vi "Check and Generate Path to Octave Executable.vi"(8 "error in (no error)":errorcluster, 11 "octave executable file or directory with executable":path=path "C:/Octave/Octave-4.0.0/bin") -> (0 "error out":errorcluster, 3 "path to exe":path)   [LabVIEW 2020, in "GOLPI library.lvlib"]
doc: "Checks path provided by user if exists. If file, consider it as Octave executable. If directory, try to look for octave-cli.exe or octave.exe. Return path to Octave executable or generate an error."
uses:
  GOLPI library.lvlib
  Custom Error Codes Enum Type Def.vi
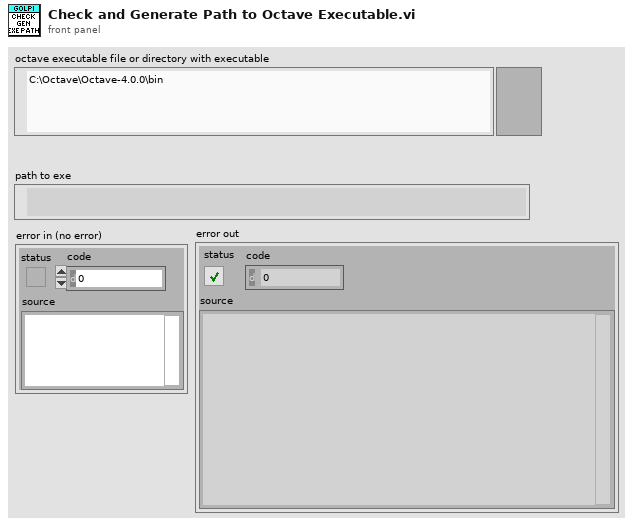
[diagram p1: front panel]
types:
  T1 = typedef "GOLPI library.lvlib/Custom Error Codes Enum Type Def.vi" = enum16{"no error", "00 working directory PAR1 missing", "01 octave binary PAR1 missing", "02 octave report error PAR1", "03 empty output last cmd PAR1", "04 missing temporary file PAR1", "05 pwd PAR 1 not exist", "06 oct package not installed", "07 octave default binary missing", "10 var PAR1 not string, vect", "11 var PAR1 not num, scal, ~compl", "12 var PAR1 not num, scal, compl", "13 var PAR1 not num, vect, ~compl", "14 var PAR1 not num, vect, compl", "15 var PAR1 not num, mat, ~compl", "16 var PAR1 not num, mat, ~compl", "30 read timeout", "60 bitstream transport failed", "61 bitstream decode error PAR1", "62 bitstream cannot be set", "70 struct transfer not possible", "80 struct: cluster elem. PAR1 not implem.", "81 struct: structure field PAR1 not implem.", "82 struct: size mismatch of PAR1", "83 struct: type mismatch of PAR1", "98 internal error", "99 not finished", "90 Not supported in Matlab mode", "91 Matlab variable transfer error", "92 Matlab Script Error"}
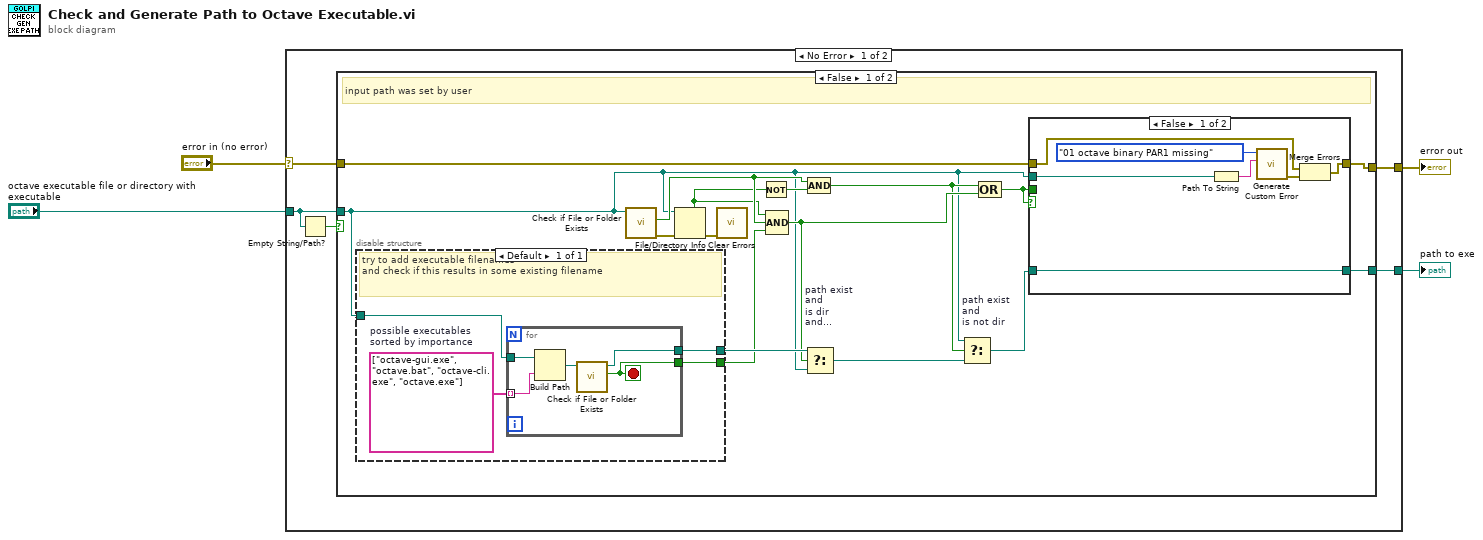
[diagram p0: block diagram]
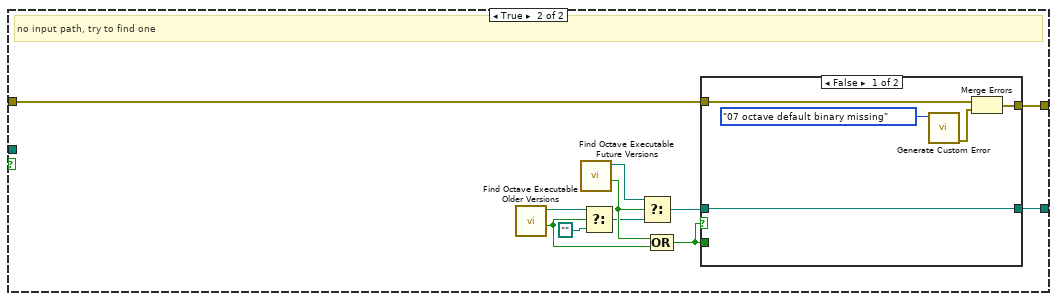
[diagram p3: hidden frame]
diagram:
  n1 = case shown="No Error" "error in (no error)" {
    selector: "error in (no error)" -> [w9 w63]
    tunnel: [w5 w63] -> w3
    tunnel: [w6 w62] -> w1
    tunnel: "octave executable file or directory with executable" -> [w8 w62]
    frame No Error {
      n2 = Empty String/Path?(string/path=w8) -> (empty?=w7:bool)
      n3 = case shown="False" w7 {
        tunnel: [w13 w47] -> w5
        tunnel: w9 -> [w14 w48]
        tunnel: [w11 w44] -> w6
        tunnel: w8 -> [w10 _]
        frame False {
          # "input path was set by user"
          n4 = disable-structure shown="Default" {
            disable-tunnel: [w28] -> w24
            disable-tunnel: [w27] -> w16
            disable-tunnel: w10 -> [w26]
            frame Enabled {
              w29 = string[] ["octave-gui.exe", "octave.bat", "octave-cli.exe", "octave.exe"]  # possible executables sorted by importance
              # "try to add executable filenames\nand check if this results in some existing filename"
              n5 = for {
                tunnel: w29 -> [w34] mode=indexing
                tunnel: w26 -> [w33]
                tunnel: [w31] -> w28
                tunnel: [w30] -> w27
                stop <- w30 stop-if-true
                n6 = Build Path(base path=w33, name or relative path=w34) -> (appended path=w32:path)
                n7 = call <vilib>:"Check if File or Folder Exists.vi"("path"=w32) -> ("file or folder exists?"=w30:bool, "dup path"=w31:path)  [unwired: 8 in, 1 out]
              }
            }
          }
          n8 = call <vilib>:"Check if File or Folder Exists.vi"("path"=w10) -> ("error out"=w25:errorcluster, "file or folder exists?"=w20:bool)  [unwired: 8 in, 1 out]
          n9 = File/Directory Info(path=w10, error in=w25) -> (directory=w19:bool, error out=w22:errorcluster)  [unwired: 5 out]
          n10 = call <vilib>:"Clear Errors.vi"("error in (no error)"=w22) -> ()  [unwired: 5 in, 2 out]
          n11 = Not(x=w19) -> (.not. x?=w21:bool)
          n12 = Compound Arithmetic op=AND(w19, w20, w16) -> (w18:bool)
          n13 = Select "path exist\nand\nis dir\nand\nexecutable found"(t=w24, s=w18, f=w10) -> (s? t:f=w23:path)
          n14 = Compound Arithmetic op=AND(w20, w21) -> (w17:bool)
          n15 = Select "path exist\nand\nis not dir"(t=w10, s=w17, f=w23) -> (s? t:f=w15:path)
          n16 = Compound Arithmetic op=OR(w17, w18) -> (w12:bool)
          n17 = case shown="False" w12 {
            tunnel: w15 -> [w36 w43]
            tunnel: w14 -> [w38 w42]
            tunnel: w12 -> [_ _]
            tunnel: [w37 w42] -> w13
            tunnel: [w36 w43] -> w11
            tunnel: w10 -> [w35 _]
            frame False {
              n18 = Path To String(path=w35) -> (string=w41:string)
              n19 = call "Generate Custom Error.vi"("PAR1"=w41, "GOLPI error"=Custom_Error_Codes_Enum_Type_Def.vi."01 octave binary PAR1 missing") -> ("error out"=w39:errorcluster)  [unwired: 9 in]
              n20 = Merge Errors(w38, w39) -> (w37:errorcluster)
            }
            frame True {
            }
          }
        }
        frame True {
          # "no input path, try to find one"
          n21 = call "Find Octave Executable Older Versions.vi"() -> ("Found executable?"=w54:bool, "Executable path"=w51:path)  [unwired: 10 in]
          n22 = call "Find Octave Executable Future Versions.vi"() -> ("Found executable?"=w53:bool, "Executable path"=w49:path)  [unwired: 10 in]
          n23 = Select(t=w51, s=w54, f=path "") -> (s? t:f=w52:path)
          n24 = Select(t=w49, s=w53, f=w52) -> (s? t:f=w45:path)
          n25 = Compound Arithmetic op=OR(w53, w54) -> (w46:bool)
          n26 = case shown="False" w46 {
            tunnel: w48 -> [w57 w60]
            tunnel: w46 -> [_ _]
            tunnel: [w56 w60] -> w47
            tunnel: [w55 w61] -> w44
            tunnel: w45 -> [w55 w61]
            frame False {
              n27 = call "Generate Custom Error.vi"("GOLPI error"=Custom_Error_Codes_Enum_Type_Def.vi."07 octave default binary missing") -> ("error out"=w58:errorcluster)  [unwired: 10 in]
              n28 = Merge Errors(w57, w58) -> (w56:errorcluster)
            }
            frame True {
            }
          }
        }
      }
    }
    frame Error {
    }
  }
  "error out" <- w3
  "path to exe" <- w1
